vi "Exit_Program_Mode.vi"(8 "error in (no error)":errorcluster, 11 "Serial Config":T1={"Baud"=9600, "Flow Ctl"=0, "Parity"=0, "COM Port"="", "Address"=1} {"Parity" items=["None", "Odd", "Even"]; "Flow Ctl" items=["None"]; "Baud" items=["4800"=4800, "9600"=9600, "19200"=19200, "38400"=38400]}) -> (0 "error out":errorcluster, 3 "Serial Config out":T1={"Baud"=9600, "Flow Ctl"=0, "Parity"=0, "COM Port"="", "Address"=0} {"Parity" items=["None", "Odd", "Even"]; "Flow Ctl" items=["None"]; "Baud" items=["4800"=4800, "9600"=9600, "19200"=19200, "38400"=38400]})   [LabVIEW 2014, in "Omega CN9600 series.lvclass"]
uses:
  Omega CN9600 series.lvclass
  Serial_Config_Omega.ctl
  <vilib>/Utility/error.llb/Error Cluster From Error Code.vi
  <vilib>/ErrorRing/Error Ring.xnode
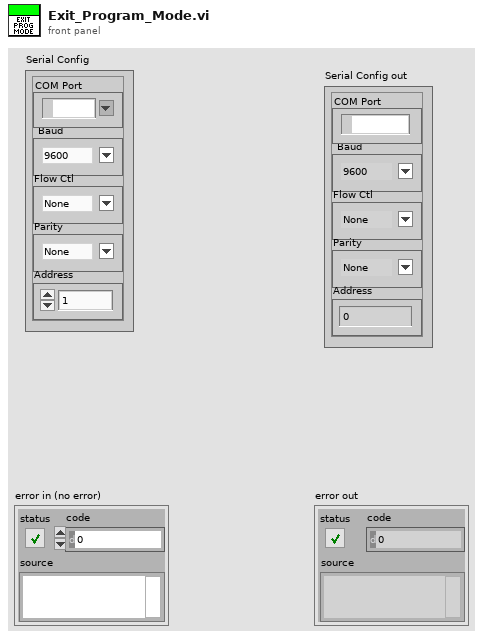
[diagram p1: front panel]
types:
  T1 = typedef "Omega CN9600 series.lvclass/Serial_Config_Omega.ctl" = cluster{"Baud":u32, "Flow Ctl":u16, "Parity":u16, "COM Port":refnum<visa-resource-name>, "Address":u8}
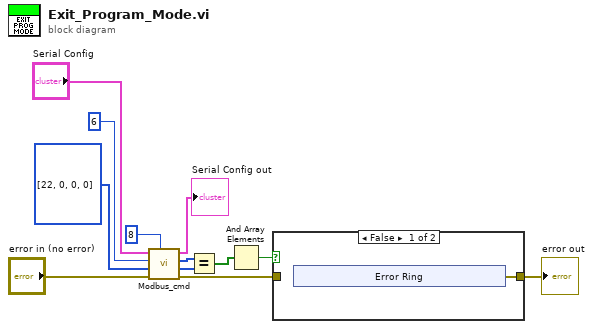
[diagram p0: block diagram]
diagram:
  n1 = call "Modbus_cmd.vi"("Bytes to read"=u32 8, "error in (no error)"="error in (no error)", "Data"=u8[] [22, 0, 0, 0], "Function"=u8 6, "Serial Config"="Serial Config") -> ("error out"=w10:errorcluster, "Cmd Sent"=w4:u8[], "Response"=w5:u8[], "Serial Config out"=→"Serial Config out":T1)  [unwired: 3 in]
  n2 = Equal?(x=w5, y=w4) -> (x = y?=w3:bool[])
  n3 = And Array Elements(Boolean array=w3) -> (logical AND=w2:bool)
  n4 = case shown="False" w2 {
    tunnel: [w13 w19] -> w11
    tunnel: w10 -> [_ w19]
    frame False {
      n5 = xnode "Error Ring"() -> ("error out"=w13:errorcluster)
    }
    frame True {
    }
  }
  "error out" <- w11
